vi "Adaptive ROI System.vi"() -> ()   [LabVIEW 2009]
uses:
  <vilib>/imath/engines/lvmath2/RunTimeEngine/ErrorHandling/NIMS_Finalize Error.vi
  <vilib>/imath/engines/lvmath2/RunTimeEngine/Parser/MC_Version.vi
  <vilib>/imath/engines/lvmath2/RunTimeEngine/NodeEndStatement/NIMS_NodeEndStatement_Output.vi
  <instcachedir>/0/NIMS_NodeEndStatement_Output_B70DDD75627E4997AAE11E9955EDAA25.lvgen/NIMS_NodeEndStatement_Output_B70DDD75627E4997AAE11E9955EDAA25_002.vi
  <instcachedir>/0/NIMS_NodeEndStatement_Output_B70DDD75627E4997AAE11E9955EDAA25.lvgen/NIMS_NodeEndStatement_Output_B70DDD75627E4997AAE11E9955EDAA25_001.vi
  <vilib>/imath/engines/lvmath/Functions/Error Handling/MergeErrorsWrapper.vi
  <vilib>/imath/engines/lvmath/Functions/Error Handling/error.ctl
  <vilib>/imath/engines/lvmath2/RunTimeEngine/BuiltInFunctions/abs/NIMS_abs(signed).vi
  <instcachedir>/0/NIMS_abs(signed)_C4FCB8E6058B49B797C7C8D53CA5F6EC.lvgen/NIMS_abs(signed)_C4FCB8E6058B49B797C7C8D53CA5F6EC_004.vi
  <instcachedir>/0/NIMS_NodeEndStatement_Output_B70DDD75627E4997AAE11E9955EDAA25.lvgen/NIMS_NodeEndStatement_Output_B70DDD75627E4997AAE11E9955EDAA25_006.vi
  <vilib>/imath/engines/lvmath/Functions/Error Handling/MC_Mask_Errors.vi
  <vilib>/imath/engines/lvmath2/RunTimeEngine/BuiltInFunctions/mean/NIMS_RRow=mean(RM,I32).vi
  <vilib>/imath/engines/lvmath2/RunTimeEngine/BuiltInFunctions/mean/NIMS_RS=mean(RV,I32).vi
  <vilib>/imathl/engines/lvmath/Functions/Error Handling/Create Error.vi
  <vilib>/imath/engines/lvmath2/RunTimeEngine/VariableToken/Read/NIMS_Get Elements - RV(_,_) - NoCheck - Check.vi
  <instcachedir>/0/NIMS_Get Elements - RV(_,_) - NoCheck - Check_2CF0E5988CCD4230910E4DE8A8D9652B.lvgen/NIMS_Get Elements - RV(_,_) - NoCheck - Check_2CF0E5988CCD4230910E4DE8A8D9652B_000.vi
  <vilib>/imath/engines/lvmath2/RunTimeEngine/RangeToken/NIMS_Range.vi
  <instcachedir>/0/NIMS_Range_6D647EC16A744C98B5DE1D649A2D648D.lvgen/NIMS_Range_6D647EC16A744C98B5DE1D649A2D648D_001.vi
  <vilib>/imath/engines/lvmath2/RunTimeEngine/VariableToken/Read/NIMS_Get Elements - RV(_) - Check(_).vi
  <instcachedir>/0/NIMS_Get Elements - RV(_) - Check(_)_82E0F2002B964B63A6FF4E3708911C3C.lvgen/NIMS_Get Elements - RV(_) - Check(_)_82E0F2002B964B63A6FF4E3708911C3C_000.vi
  <instcachedir>/0/NIMS_Range_6D647EC16A744C98B5DE1D649A2D648D.lvgen/NIMS_Range_6D647EC16A744C98B5DE1D649A2D648D_000.vi
  <vilib>/imath/engines/lvmath2/RunTimeEngine/BuiltInFunctions/max/1 input/NIMS_max(RV).vi
  <instcachedir>/0/NIMS_max(RV)_2C608606CE4049CAAC45B6670A7A9B83.lvgen/NIMS_max(RV)_2C608606CE4049CAAC45B6670A7A9B83_000.vi
  <vilib>/imath/engines/lvmath2/RunTimeEngine/BuiltInFunctions/is_nan/NIMS_is_nan.vi
  <instcachedir>/0/NIMS_is_nan_83F2CBA22B22468D9582265D5B29A05F.lvgen/NIMS_is_nan_83F2CBA22B22468D9582265D5B29A05F_000.vi
  <vilib>/imath/engines/lvmath2/RunTimeEngine/VariableToken/Read/NIMS_Get Elements - RV(_) - Check.vi
  <instcachedir>/0/NIMS_Get Elements - RV(_) - Check_60F12861D0564803969A5D0D0D1716CD.lvgen/NIMS_Get Elements - RV(_) - Check_60F12861D0564803969A5D0D0D1716CD_002.vi
  <vilib>/imath/engines/lvmath2/RunTimeEngine/ReplaceToken/NIMS_Replace - V(S)=S.vi
  <instcachedir>/0/NIMS_Replace - V(S)=S_670A9E0533664C1D848C8E58B3321B6A.lvgen/NIMS_Replace - V(S)=S_670A9E0533664C1D848C8E58B3321B6A_000.vi
  <vilib>/imath/engines/lvmath2/RunTimeEngine/ReplaceToken/NIMS_Replace - Size Check _(_)=S.vi
  <instcachedir>/0/NIMS_Replace - Size Check _(_)=S_8596181D73404097BAB9CBB006194BB0.lvgen/NIMS_Replace - Size Check _(_)=S_8596181D73404097BAB9CBB006194BB0_000.vi
  <vilib>/imath/engines/lvmath2/RunTimeEngine/ReplaceToken/NIMS_Replace - Check Linear.vi
  <instcachedir>/0/NIMS_Replace - Check Linear_9243CBB174894FF6977027453DA6955E.lvgen/NIMS_Replace - Check Linear_9243CBB174894FF6977027453DA6955E_001.vi
  <vilib>/imath/engines/lvmath2/RunTimeEngine/CommandStatement/MC_CommandStatement_break.vi
  <vilib>/imath/engines/lvmath2/RunTimeEngine/BuiltInFunctions/size/NIMS_[I32,I32]=size(GM).vi
  <instcachedir>/0/NIMS_[I32,I32]=size(GM)_B0A6EC1255BB4C8AB801FE6F734128D9.lvgen/NIMS_[I32,I32]=size(GM)_B0A6EC1255BB4C8AB801FE6F734128D9_000.vi
  <instcachedir>/0/NIMS_abs(signed)_C4FCB8E6058B49B797C7C8D53CA5F6EC.lvgen/NIMS_abs(signed)_C4FCB8E6058B49B797C7C8D53CA5F6EC_003.vi
  <vilib>/imath/engines/lvmath2/RunTimeEngine/VariableToken/NIMS_VariableToken_CondDefined.vi
  <instcachedir>/0/NIMS_VariableToken_CondDefined_5641E79000FB4D628475532441475385.lvgen/NIMS_VariableToken_CondDefined_5641E79000FB4D628475532441475385_000.vi
  <vilib>/imath/engines/lvmath2/RunTimeEngine/VariableToken/Read/NIMS_Get Elements - SorM(_,_) - Check(_) - Check(_).vi
  <instcachedir>/0/NIMS_Get Elements - SorM(_,_) - Check(_) - Check(_)_765307169EBF4B10AFB614967F0850B3.lvgen/NIMS_Get Elements - SorM(_,_) - Check(_) - Check(_)_765307169EBF4B10AFB614967F0850B3_000.vi
  <vilib>/imath/engines/lvmath/Functions/Error Handling/MC_Error Cluster From Error Code.vi
  <instcachedir>/0/NIMS_abs(signed)_C4FCB8E6058B49B797C7C8D53CA5F6EC.lvgen/NIMS_abs(signed)_C4FCB8E6058B49B797C7C8D53CA5F6EC_002.vi
  <vilib>/imath/engines/lvmath2/RunTimeEngine/BuiltInFunctions/fftshift/NIMS_fftshift(GM).vi
  <instcachedir>/0/NIMS_fftshift(GM)_854644D58B904BE68890FF38C728418A.lvgen/NIMS_fftshift(GM)_854644D58B904BE68890FF38C728418A_000.vi
  <vilib>/imath/engines/lvmath2/RunTimeEngine/BuiltInFunctions/fft2d/NIMS_fft2d.vi
  <instcachedir>/0/NIMS_fft2d_5F3590B2E5BC4AF3BD6395730A2DC379.lvgen/NIMS_fft2d_5F3590B2E5BC4AF3BD6395730A2DC379_000.vi
  <vilib>/imath/engines/lvmath2/RunTimeEngine/BuiltInFunctions/meshgrid2d/NIMS_meshgrid2d(V,V).vi
  <instcachedir>/0/NIMS_meshgrid2d(V,V)_E4FD91C5AC284970A2AC10945542E876.lvgen/NIMS_meshgrid2d(V,V)_E4FD91C5AC284970A2AC10945542E876_000.vi
  <vilib>/imath/engines/lvmath2/RunTimeEngine/BuiltInFunctions/cart_to_polar/NIMS_cart_to_polar(M3).vi
  <vilib>/imath/engines/lvmath2/RunTimeEngine/BuiltInFunctions/round/NIMS_round(DBL).vi
  <vilib>/imath/engines/lvmath2/RunTimeEngine/BuiltInFunctions/zeros/NIMS_V=zeros(I32,I32).vi
  <vilib>/imath/engines/lvmath2/RunTimeEngine/ReplaceToken/NIMS_Replace - Assignment Check _(_)=VorM.vi
  <instcachedir>/0/NIMS_Replace - Assignment Check _(_)=VorM_092AB1ED6AF9404A81BC0E556665BBDA.lvgen/NIMS_Replace - Assignment Check _(_)=VorM_092AB1ED6AF9404A81BC0E556665BBDA_001.vi
  <vilib>/imath/engines/lvmath2/RunTimeEngine/ReplaceToken/NIMS_Replace - Size Check _(_)=VorM.vi
  <instcachedir>/0/NIMS_Replace - Size Check _(_)=VorM_5D763D18DEEF46AFB676FCB035E69D92.lvgen/NIMS_Replace - Size Check _(_)=VorM_5D763D18DEEF46AFB676FCB035E69D92_001.vi
  <vilib>/imath/engines/lvmath2/RunTimeEngine/VariableToken/Read/NIMS_Get Elements - SorM(_) - Check.vi
  <instcachedir>/0/NIMS_Get Elements - SorM(_) - Check_7ED6A6929A794478AD00936E11BC64AA.lvgen/NIMS_Get Elements - SorM(_) - Check_7ED6A6929A794478AD00936E11BC64AA_000.vi
  <vilib>/imath/engines/lvmath2/RunTimeEngine/BuiltInFunctions/findnz/NIMS_[1o]_findnz(GM).vi
  <instcachedir>/0/NIMS_[1o]_findnz(GM)_DBE08F0D46E742F4956471D0BFAB2CB2.lvgen/NIMS_[1o]_findnz(GM)_DBE08F0D46E742F4956471D0BFAB2CB2_000.vi
  <instcachedir>/0/NIMS_Replace - Assignment Check _(_)=VorM_092AB1ED6AF9404A81BC0E556665BBDA.lvgen/NIMS_Replace - Assignment Check _(_)=VorM_092AB1ED6AF9404A81BC0E556665BBDA_000.vi
  <instcachedir>/0/NIMS_Replace - Size Check _(_)=VorM_5D763D18DEEF46AFB676FCB035E69D92.lvgen/NIMS_Replace - Size Check _(_)=VorM_5D763D18DEEF46AFB676FCB035E69D92_000.vi
  <instcachedir>/0/NIMS_Replace - Check Linear_9243CBB174894FF6977027453DA6955E.lvgen/NIMS_Replace - Check Linear_9243CBB174894FF6977027453DA6955E_000.vi
  <vilib>/imath/engines/lvmath2/RunTimeEngine/BuiltInFunctions/polyfit/NIMS_[2o]_polyfit.vi
  <vilib>/imath/engines/lvmath2/RunTimeSupport/NIMS_Complex To Real.vi
  <instcachedir>/0/NIMS_Complex To Real_7B9C6496820F433C8523AD0145A83A8A.lvgen/NIMS_Complex To Real_7B9C6496820F433C8523AD0145A83A8A_000.vi
  <vilib>/imath/engines/lvmath2/RunTimeEngine/VariableToken/NIMS_VariableToken_CondDefinedDefinedByReplace.vi
  <instcachedir>/0/NIMS_VariableToken_CondDefinedDefinedByReplace_D162CFFC24174562A9FEA619A91E1A56.lvgen/NIMS_VariableToken_CondDefinedDefinedByReplace_D162CFFC24174562A9FEA619A91E1A56_000.vi
  <instcachedir>/0/NIMS_abs(signed)_C4FCB8E6058B49B797C7C8D53CA5F6EC.lvgen/NIMS_abs(signed)_C4FCB8E6058B49B797C7C8D53CA5F6EC_001.vi
  <vilib>/imath/engines/lvmath2/RunTimeEngine/BuiltInFunctions/min/1 input/NIMS_min(RV).vi
  <instcachedir>/0/NIMS_min(RV)_AE994CF480B345CA9E0CB3DC5B6A3F66.lvgen/NIMS_min(RV)_AE994CF480B345CA9E0CB3DC5B6A3F66_000.vi
  <instcachedir>/0/NIMS_abs(signed)_C4FCB8E6058B49B797C7C8D53CA5F6EC.lvgen/NIMS_abs(signed)_C4FCB8E6058B49B797C7C8D53CA5F6EC_000.vi
  <vilib>/imath/engines/lvmath2/RunTimeEngine/BuiltInFunctions/rem/NIMS_rem_no checks.vi
  <instcachedir>/0/NIMS_rem_no checks_4CC9B305AB7E42EF90AFC4973FB32F8D.lvgen/NIMS_rem_no checks_4CC9B305AB7E42EF90AFC4973FB32F8D_000.vi
  <vilib>/imath/engines/lvmath2/RunTimeEngine/BuiltInFunctions/size/NIMS_I32Row=size(GM).vi
  <instcachedir>/0/NIMS_I32Row=size(GM)_10ACDCB9F1F84A7E9F42C91D87611FB5.lvgen/NIMS_I32Row=size(GM)_10ACDCB9F1F84A7E9F42C91D87611FB5_000.vi
  <instcachedir>/0/NIMS_NodeEndStatement_Output_B70DDD75627E4997AAE11E9955EDAA25.lvgen/NIMS_NodeEndStatement_Output_B70DDD75627E4997AAE11E9955EDAA25_005.vi
  <instcachedir>/0/NIMS_Get Elements - RV(_) - Check_60F12861D0564803969A5D0D0D1716CD.lvgen/NIMS_Get Elements - RV(_) - Check_60F12861D0564803969A5D0D0D1716CD_001.vi
  <vilib>/imath/engines/lvmath2/RunTimeEngine/BuiltInFunctions/conv2d/NIMS_conv2d(GM,GM,Str).vi
  <instcachedir>/0/NIMS_conv2d(GM,GM,Str)_C7D81E1B98E043D08C3460674E88E962.lvgen/NIMS_conv2d(GM,GM,Str)_C7D81E1B98E043D08C3460674E88E962_001.vi
  <vilib>/imath/engines/lvmath2/RunTimeEngine/ArithmeticOperatorToken/NIMS_ArithmeticOperator_plus.vi
  <instcachedir>/0/NIMS_ArithmeticOperator_plus_C2557ADBC1AF4CC89A8D103312A7892D.lvgen/NIMS_ArithmeticOperator_plus_C2557ADBC1AF4CC89A8D103312A7892D_002.vi
  <vilib>/imath/engines/lvmath2/RunTimeEngine/BuiltInFunctions/sum/NIMS_sum(GM,Sca).vi
  <instcachedir>/0/NIMS_sum(GM,Sca)_1EB0DF48B4224309BC0660E7CC5423AB.lvgen/NIMS_sum(GM,Sca)_1EB0DF48B4224309BC0660E7CC5423AB_000.vi
  <vilib>/imath/engines/lvmath2/RunTimeEngine/VariableToken/Read/NIMS_Get Elements - SorM(_,_) - Check - Check.vi
  <instcachedir>/0/NIMS_Get Elements - SorM(_,_) - Check - Check_48F983ECF9704C8392806B5FDD2F5E51.lvgen/NIMS_Get Elements - SorM(_,_) - Check - Check_48F983ECF9704C8392806B5FDD2F5E51_001.vi
  <vilib>/imath/engines/lvmath2/RunTimeEngine/BuiltInFunctions/sum/NIMS_sum(GV).vi
  <instcachedir>/0/NIMS_sum(GV)_6582ACC3CFD94C22B1CA3BD4A8C5E9ED.lvgen/NIMS_sum(GV)_6582ACC3CFD94C22B1CA3BD4A8C5E9ED_000.vi
  <instcachedir>/0/NIMS_Get Elements - RV(_) - Check_60F12861D0564803969A5D0D0D1716CD.lvgen/NIMS_Get Elements - RV(_) - Check_60F12861D0564803969A5D0D0D1716CD_000.vi
  <vilib>/imath/engines/lvmath2/RunTimeEngine/VariableToken/Read/NIMS_Get Elements - CV(_) - Check.vi
  <instcachedir>/0/NIMS_Get Elements - CV(_) - Check_BEC96A94B22A447C8D443292564CBCD4.lvgen/NIMS_Get Elements - CV(_) - Check_BEC96A94B22A447C8D443292564CBCD4_000.vi
  <vilib>/imath/engines/lvmath2/RunTimeEngine/ReplaceToken/NIMS_Replace - M(#,S)=S.vi
  <instcachedir>/0/NIMS_Replace - M(#,S)=S_1219E6139A4243FF9F5238A5EFF7E472.lvgen/NIMS_Replace - M(#,S)=S_1219E6139A4243FF9F5238A5EFF7E472_001.vi
  <vilib>/imath/engines/lvmath2/RunTimeEngine/ReplaceToken/NIMS_Replace - Size Check M(#,_)=S.vi
  <instcachedir>/0/NIMS_Replace - Size Check M(#,_)=S_E9F0A723BCFB4C07851EF854435358BF.lvgen/NIMS_Replace - Size Check M(#,_)=S_E9F0A723BCFB4C07851EF854435358BF_001.vi
  <vilib>/imath/engines/lvmath2/RunTimeEngine/ReplaceToken/NIMS_Replace - Check(_) Column.vi
  <instcachedir>/0/NIMS_Replace - Check(_) Column_2F70AC15C33C40AE8160DC5A87C7C261.lvgen/NIMS_Replace - Check(_) Column_2F70AC15C33C40AE8160DC5A87C7C261_003.vi
  <vilib>/imath/engines/lvmath2/RunTimeEngine/Managers/WorkSpace/UID Generator.vi
  <instcachedir>/0/NIMS_NodeEndStatement_Output_B70DDD75627E4997AAE11E9955EDAA25.lvgen/NIMS_NodeEndStatement_Output_B70DDD75627E4997AAE11E9955EDAA25_007.vi
  <vilib>/imath/engines/lvmath2/RunTimeEngine/Managers/SymbolTable/Clear UID.vi
  <vilib>/imath/engines/lvmath2/RunTimeEngine/LocalVariableDefStatement/MC_LocalVariableDefStatement_Display.vi
  <vilib>/imath/engines/lvmath2/RunTimeEngine/RunTimeType/NIMS_RunTimeType_From StrictType (excl LVString).vi
  <instcachedir>/0/NIMS_ArithmeticOperator_plus_C2557ADBC1AF4CC89A8D103312A7892D.lvgen/NIMS_ArithmeticOperator_plus_C2557ADBC1AF4CC89A8D103312A7892D_001.vi
  <vilib>/imath/engines/lvmath2/RunTimeEngine/VariableToken/Read/NIMS_Get Elements - SorM(#,_) - Check(_).vi
  <instcachedir>/0/NIMS_Get Elements - SorM(#,_) - Check(_)_3C902678D53E40FDBC79E118A936F6E4.lvgen/NIMS_Get Elements - SorM(#,_) - Check(_)_3C902678D53E40FDBC79E118A936F6E4_000.vi
  <vilib>/vision/NI_Vision_Development_Module.lvlib
  <vilib>/imath/engines/lvmath2/RunTimeEngine/Managers/SymbolTable/NIMS_WorkSpace.lvlib
panel:
  in  "AVI file to play":path
  out "focus":dbl[](array[numeric])
  out "edge":dbl[](array[numeric])
  out "motion":dbl[](array[numeric])
  out "Frame #":dbl
  out "Edge Detectives 2":dbl[](array[numeric])
  out "Image 4":T1(plugin-control)
  in  "Threshold 2":dbl=125.0
  out "Image 2":T1(plugin-control)
  in  "% thru movie":dbl(slide) scale=0.0..95.0
  out "Frame Width":dbl
  out "Frame height":dbl
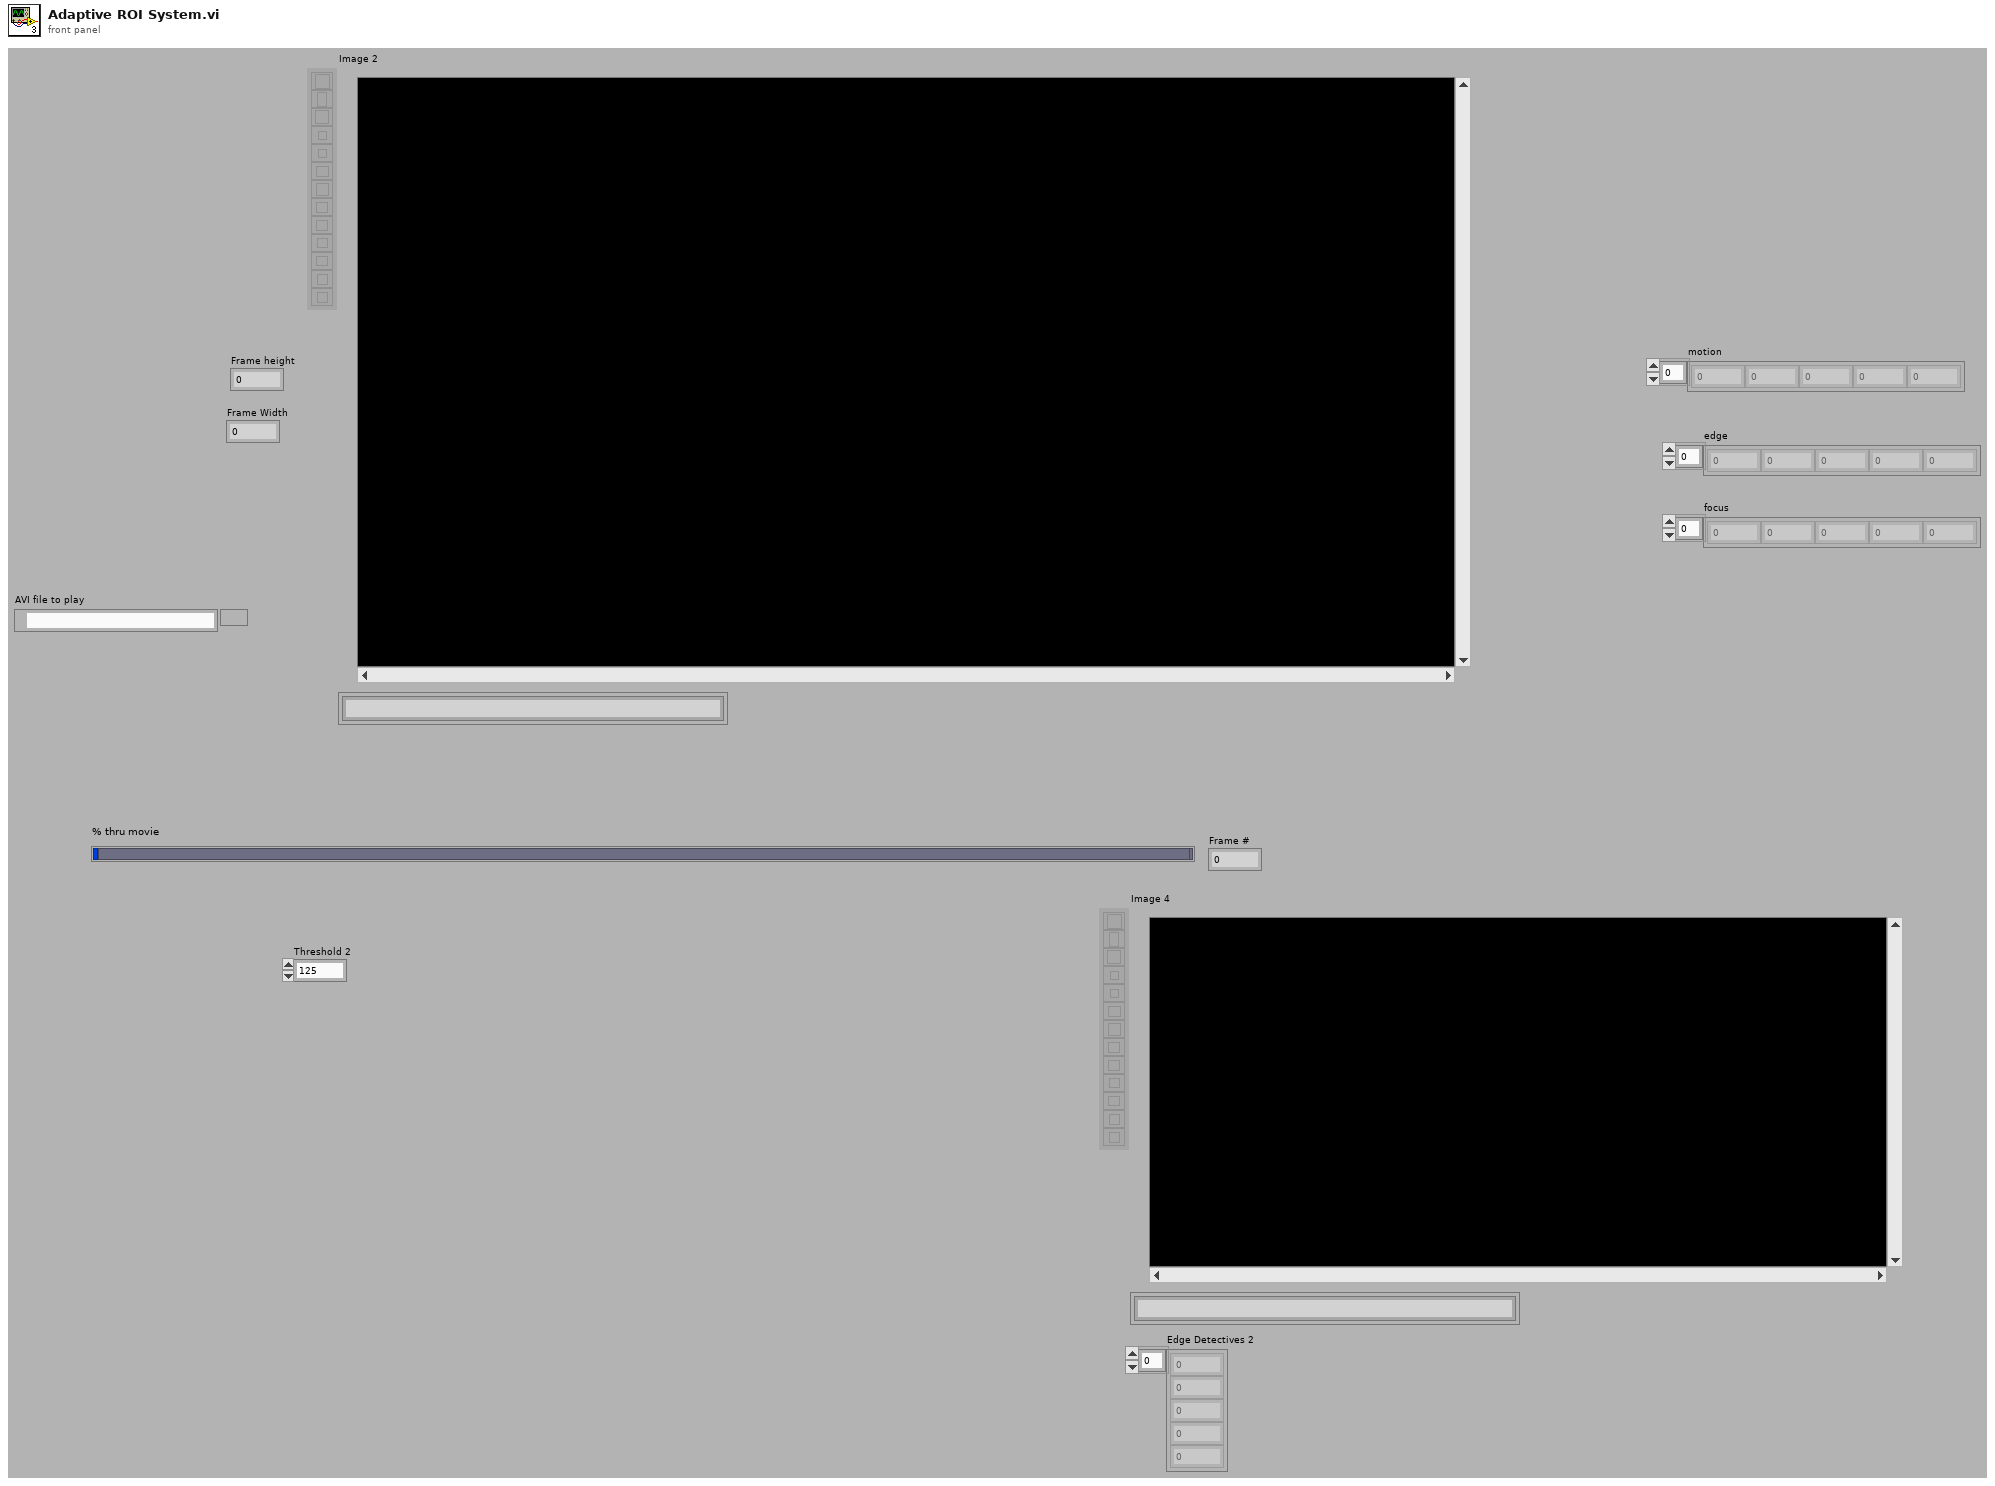
[diagram p1: front panel]
types:
  T1 = typedef "IMAQ Image.ctl" = refnum<image>
  T2 = typedef "AviRefnum.ctl" = refnum<k1>
  T3 = typedef "Image Type" = u32
  T4 = cluster{"width":u32, "height":u32, "framesPerSecond":u32, "compressionFilter":string, "hasData":bool}
  T5 = typedef "error.ctl" = enum16{"No Error", "Problem", "Unused002", "Incorrect number of parameters", "Function not defined for non-numeric types", "Unused005", "Function only defined for character arrays", "Function not defined for boolean, character, or single precision", "Function not defined for complex types", "Not a valid operation", "Inputs must be scalar", "Input matrices are not the same size", "Unused012", "Input matrices must be nonnegative integers of the same type", "Arguments must be non-negative integers less than bitmax", "Number to complement must be less than 2^N", "Bit to get is outside range", "Bit to set is outside range", "Input must be real type ", "At least one parameter must be scalar", "Unused020", "Function not defined for\nhigher dimensional matrices.", "Invalid attributes", "Wrong Type of Input Arguments", "Wrong Argument Option", "Unused025", "Indices must be real positive integers", "Unused027", "Number of elements must be the same for indices and values", "Unused029", "Cannot resize a 2D matrix with a linear index", "Unknown variable or symbol", "Indices out of range", "Empty matrix deletion can not be used with two indices", "Number of rows and columns must be the same for indices and values.", "Complex cannot be converted to Boolean", "Char cannot be converted to Boolean", "int64 cannot be converted to Boolean", "uint64 cannot be converted to Boolean", "Unused039", "Unused040", "All rows must have the same number of columns", "Incompatible types", "Invalid matrix dimensions", "Dimension must be 1 or 2", "Base must be an integer between 2 and 36", "Invalid input", "Square matrix required", "Function 'timerstart' must be called before 'timerstop'", "Arguments must be positive real", "Step must not be zero", "Wrong number of input arguments", "Wrong number of output arguments", "Unused053", "Input scalar must be >= 0", "Input scalar must be positive", "Input scalar must not be 0", "Input scalar must be in range [0,1]", "Unused058", "Input must be a vector", "Unused060", "Empty vector error", "All elements must be in domain [-1,1]", "All real elements of input vector must be >= 0", "All elements of input vector must be positive", "Values of input vectors are not compatible", "Unused066", "Input vector must be an increasing vector", "Unused068", "Unused069", "Lenths of two input vectors are not compatible", "Unused071", "Empty matrix error", "Unused073", "Unused074", "Unused075", "Unused076", "Unused077", "Size of input matrix is incompatible with input size", "Invalid format specifier", "Unused080", "Unused081", "Unused082", "Unused083", "Unused084", "Unused085", "RunTime: MathScript could not be compiled", "Unknown function", "Only scalars and strings supported", "Unused089", "Unused090", "Range is too large", "End used without variable", "Function not available (RTE)", "Custom user error", "Arguments must be integers less than bitmax", "Shared library not found", "Header file not found", "Shared library already loaded", "Shared library not loaded", "Shared library function not found", "Shared library string return problem", "Problem calling shared library function", "Problem loading shared library from OS", "Problem parsing shared library header file", "Shared library incompatible types", "Shared library unsupported return type", "Shared library function not exported", "Shared library unsupported input type", "Problem unloading shared library from OS", "Function only available from UI", "Invalid function specified in argument", "An internal error has occurred", "Invalid object", "Invalid property", "Read-only property", "A break command has occurred", "A continue command has occurred", "A return command has occurred", "ode: times parameter invalid", "Unused120", "Function not found in file", "Reserved keyword cannot be defined as variable", "Reserved keyword cannot be defined as a function or script", "Arguments must be string literals", "Function not supported on this platform", "All columns must have the same number of rows", "Function ignored in RTE warning", "Cannot use : as a parameter that is not a variable", "Output can't be coerced to requested type", "Function not supported on current target", "Variable dependent on an unwired function input", "Unused132", "Unused133", "Unused134", "Unused135", "Unused136", "Unused137", "Unused138", "Unused139", "Unused140", "Unused141", "Unused142", "Unused143", "Unused144", "Unused145", "Unused146", "MathScript parser DLL missing", "MathScript requires LabVIEW Full", "MathScript license is invalid or missing"}
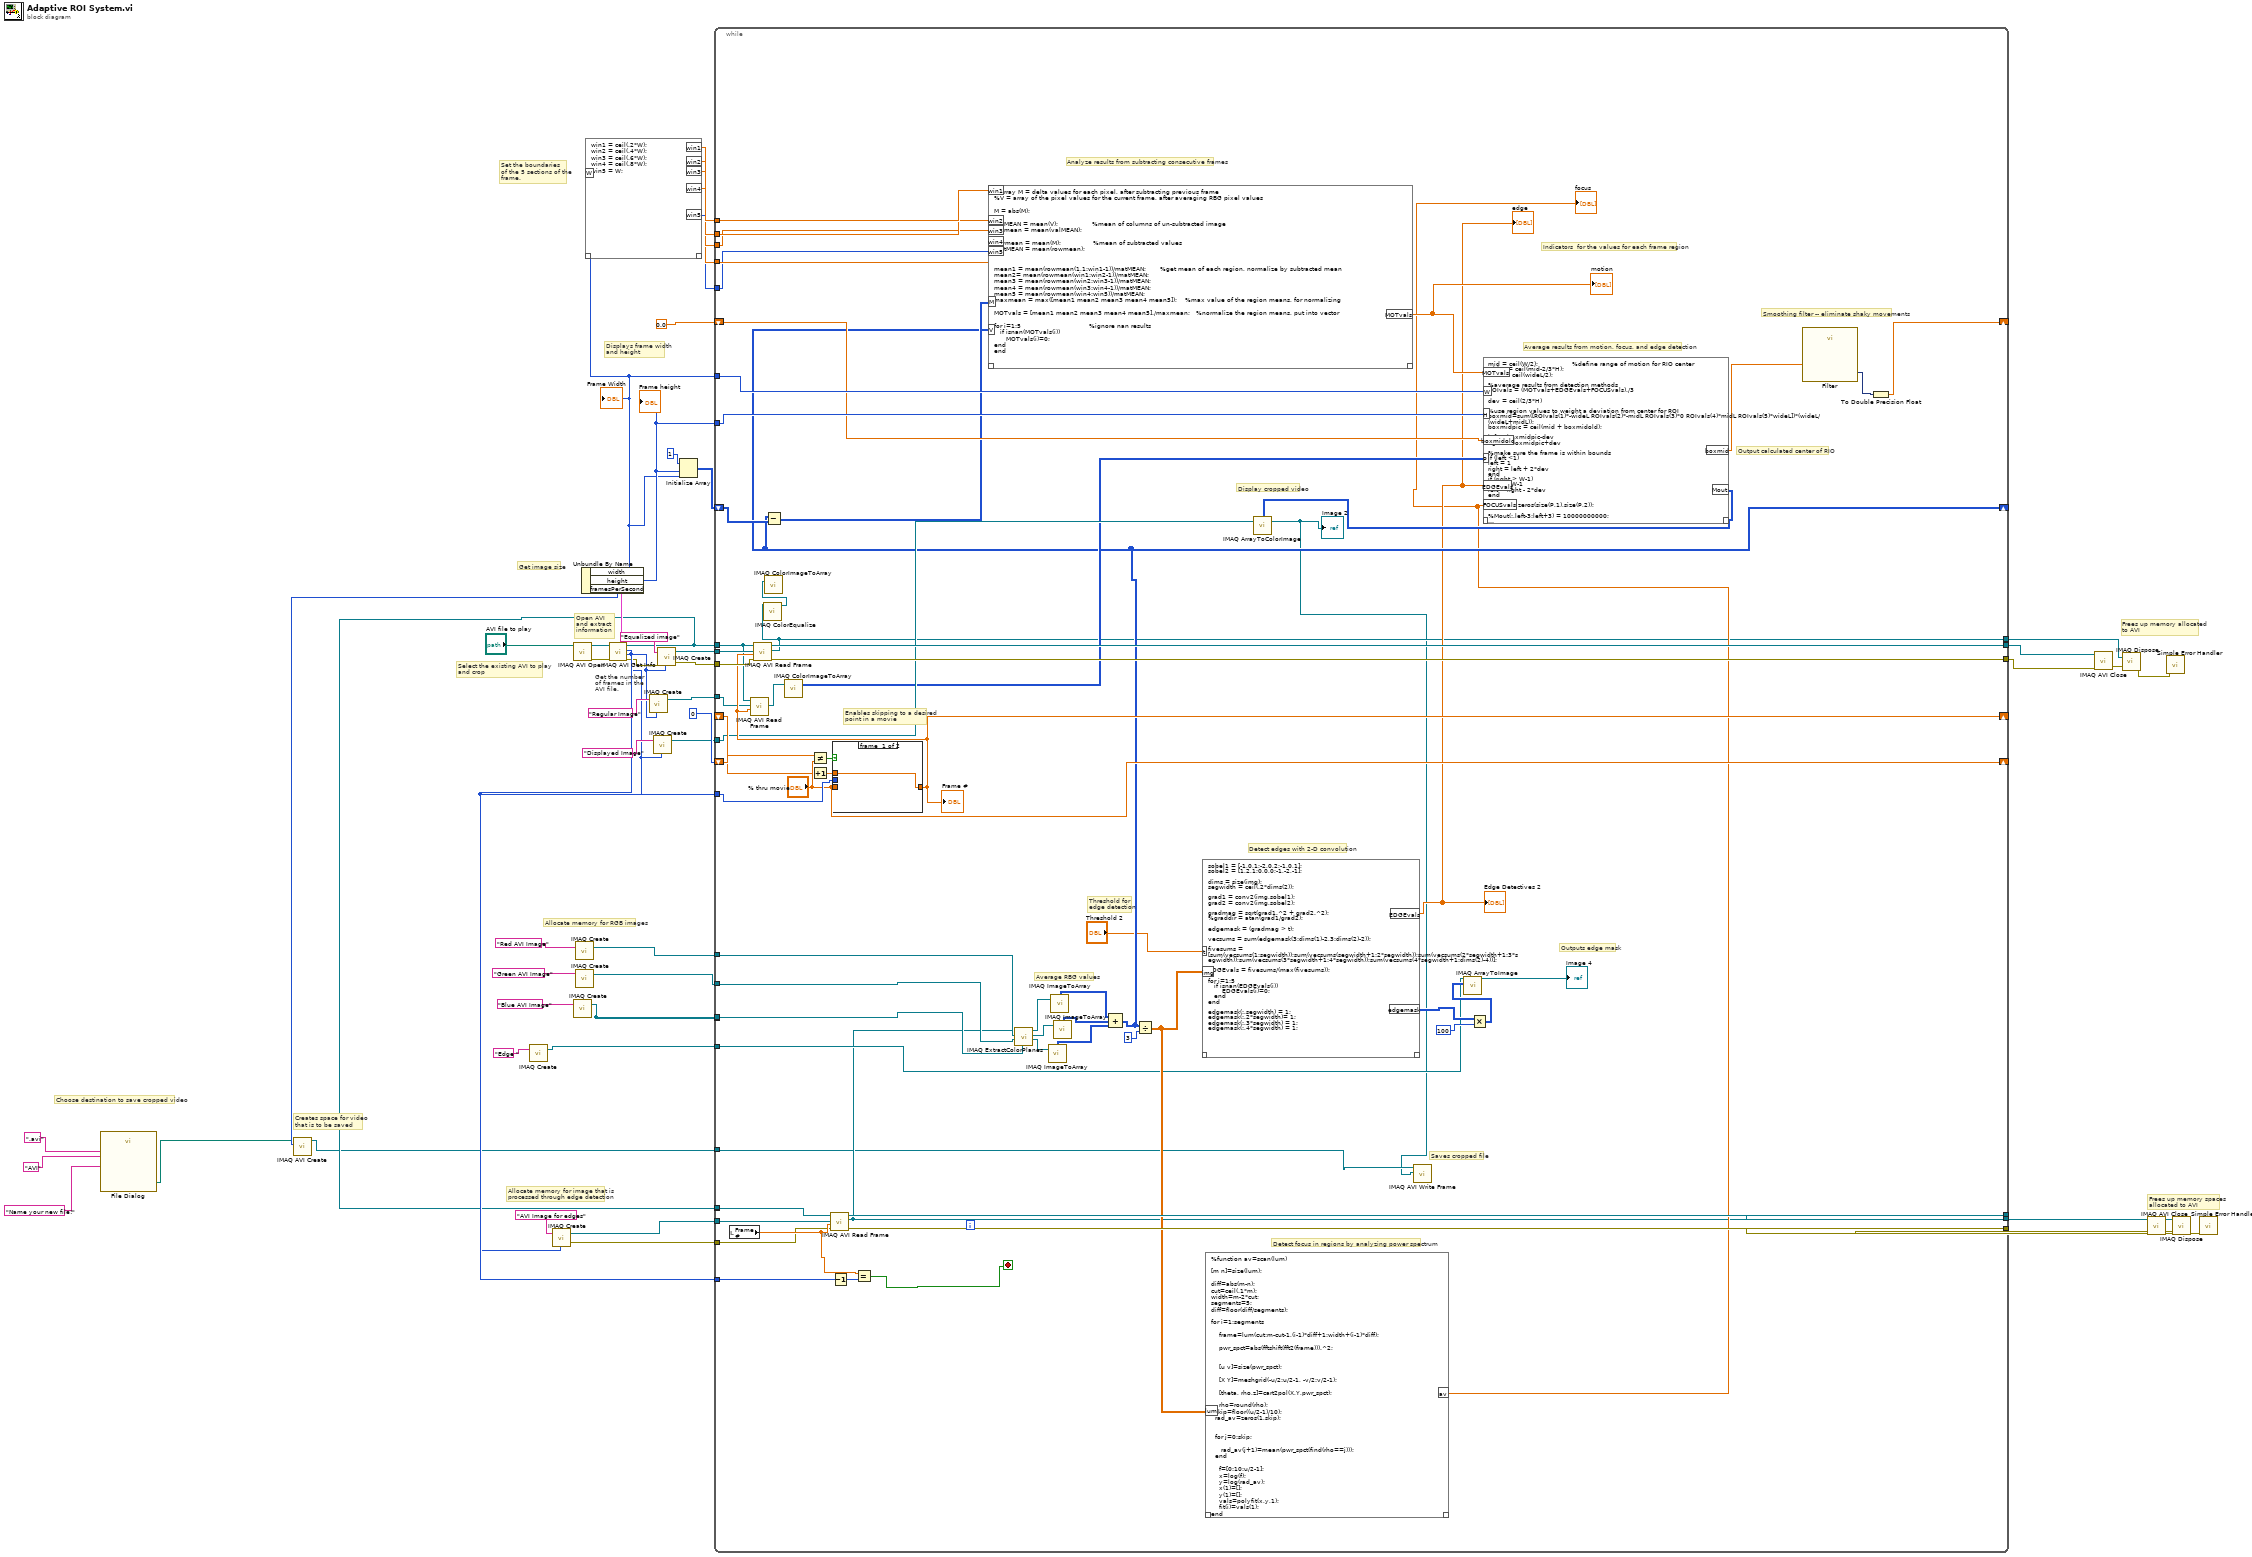
[diagram p0: block diagram]
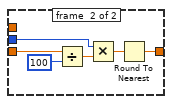
[diagram p2: hidden frame]
diagram:
  # "Creates space for video\nthat is to be saved"
  # "Displays frame width\nand height"
  # "Frees up memory allocated\nto AVI"
  # "Frees up memory spaces\nallocated to AVI"
  # "Open AVI and extract information"
  # "Allocate memory for image that is \nprocessed through edge detection"
  # "Get image size"
  # "Set the boundaries\nof the 5 sections of the\nframe."
  # "Select the existing AVI to play\nand crop"
  # "Allocate memory for RGB images"
  # "Choose destination to save cropped video"
  # "Get the number\nof frames in the\nAVI file."
  n1 = call "File Dialog"("prompt"="Name your new file!", "pattern (all files)"=".avi", "pattern label"="AVI") -> ("selected path"=w2:path)  [unwired: 9 in, 3 out]
  n2 = call "IMAQ Create"("Image Name"="Edge ") -> ("New Image"=w21:T1)  [unwired: 4 in, 1 out]
  n3 = call "IMAQ AVI Open"("AVI Path"="AVI file to play") -> ("error out"=w50:errorcluster, "Avi Refnum"=w49:T2)  [unwired: 1 in, 8 out]
  n4 = call "IMAQ Create"("Image Name"="Blue AVI Image") -> ("New Image"=w22:T1)  [unwired: 4 in, 1 out]
  n5 = call "IMAQ Create"("Image Name"="Red AVI Image") -> ("New Image"=w24:T1)  [unwired: 4 in, 1 out]
  n6 = call "IMAQ Create"("Image Name"="Green AVI Image") -> ("New Image"=w23:T1)  [unwired: 4 in, 1 out]
  n7 = call "IMAQ AVI Get Info"("error in (no error)"=w50, "Avi Refnum"=w49) -> ("error out"=w4:errorcluster, "Image Type"=w3:T3, "Number of Frames"=w20:u32, "Avi Refnum (duplicate)"=w18:T2, "Frame Data"=w51:T4)  [unwired: 5 out]
  n8 = call "IMAQ Create"("Image Name"="AVI Image for edges", "Image Type"=w3) -> ("New Image"=w19:T1, "error out"=w16:errorcluster)  [unwired: 2 in, 1 out]
  n9 = Unbundle By Name(w51) -> ("width"=w30:u32, "height"=w36:u32, "framesPerSecond"=w5:u32)
  "Frame height" <- w36
  "Frame Width" <- w30
  n10 = call "IMAQ AVI Create"("Frames Per Second"=w5, "AVI Path"=w2) -> ("Avi Refnum"=w11:T2)  [unwired: 8 in, 1 out]
  n11 = mathscript code="win1 = ceil(.2*W);\nwin2 = ceil(.4*W);\nwin3 = ceil(.6*W);\nwin4 = ceil(.8*W);\nwin5 = W;"("W"=w30) -> ("win1"=w35:dbl, "win2"=w34:dbl, "win3"=w33:dbl, "win4"=w32:dbl, "win5"=w31:u32)  [unwired: 1 in, 1 out]
  n12 = call "IMAQ Create"("Image Name"="Regular Image", "Image Type"=w3) -> ("New Image"=w39:T1)  [unwired: 3 in, 1 out]
  n13 = call "IMAQ Create"("Image Name"="Displayed Image", "Image Type"=w3) -> ("New Image"=w37:T1)  [unwired: 3 in, 1 out]
  n14 = call "IMAQ Create"("Image Name"="Equalized image", "Image Type"=w3, "error in (no error)"=w4) -> ("New Image"=w46:T1, "error out"=w15:errorcluster)  [unwired: 1 in, 1 out]
  n15 = Initialize Array(1, w36, w30) -> (w42:i32[][])
  n16 = while {
    tunnel: w46 -> [w117]
    tunnel: [w118] -> w47
    tunnel: [w116] -> w48
    tunnel: w18 -> [w106]
    tunnel: [w61] -> w44
    tunnel: w15 -> [w115]
    shift-right: [w68] -> _
    shift-left: w42 -> [w108]
    tunnel: w20 -> [w112]
    shift-right: ["% thru movie"] -> _
    shift-left: 0 -> [w114]
    shift-right: [w107] -> _
    shift-left: _ -> [w110]
    tunnel: w39 -> [w60]
    tunnel: w37 -> [w105]
    tunnel: w30 -> [w74]
    tunnel: w36 -> [w73]
    tunnel: w35 -> [w104]
    tunnel: w34 -> [w103]
    tunnel: w33 -> [w102]
    tunnel: w32 -> [w101]
    tunnel: w31 -> [w100]
    shift-right: [w98] -> _
    shift-left: 0.0 -> [w72]
    tunnel: w24 -> [w87]
    tunnel: w23 -> [w86]
    tunnel: w22 -> [_]
    tunnel: w22 -> [w85]
    tunnel: w21 -> [w58]
    tunnel: w20 -> [w83]
    tunnel: w19 -> [w80]
    tunnel: [w79] -> _
    tunnel: w18 -> [w79]
    tunnel: w16 -> [w78]
    tunnel: w11 -> [w55]
    tunnel: [w77] -> w10
    tunnel: [w57] -> w8
    tunnel: [w76] -> w9
    stop <- w81 stop-if-true
    # "Threshold for \nedge detection"
    # "Enables skipping to a desired\npoint in a movie"
    # "Saves cropped file"
    # "Outputs edge mask"
    # "Detect focus in regions by analyzing power spectrum"
    # "Average RBG values"
    # "Detect edges with 2-D convolution"
    # "Display cropped video"
    # "Output calculated center of RIO"
    # "Average results from motion, focus, and edge detection"
    # "Smoothing filter -- eliminate shaky movements"
    # "Indicators  for the values for each frame region"
    # "Analyze results from subtracting consecutive frames"
    n17 = local read "Frame #"() -> (w82:dbl)
    n18 = Not Equal?(x=w114, y="% thru movie") -> (x != y?=w113:bool)
    n19 = Increment(x=w110) -> (x+1=w109:dbl)
    n20 = call "IMAQ AVI Read Frame"("error in (no error)"=w78, "Frame Number"=w82, "Image"=w80, "Avi Refnum"=w79) -> ("error out"=w77:errorcluster, "Image Out"=w57:T1, "Avi Refnum (duplicate)"=w76:T2)  [unwired: 1 in, 4 out]
    n21 = Decrement(x=w83) -> (x-1=w84:u32)
    n22 = case shown="True" w113 {
      tunnel: "% thru movie" -> [_ w1788]
      tunnel: w112 -> [_ w1791]
      tunnel: [w1785 w1789] -> w107
      tunnel: w109 -> [w1785 _]
      frame #0 {
      }
      frame #1 {
        n23 = Divide(x=w1788, y=100) -> (x/y=w1786:dbl)
        n24 = Multiply(x=w1791, y=w1786) -> (x*y=w1790:dbl)
        n25 = Round To Nearest(number=w1790) -> (nearest integer value=w1789:dbl)
      }
    }
    "Frame #" <- w107
    n26 = call "IMAQ AVI Read Frame"("Frame Number"=w107, "Image"=w60, "Avi Refnum"=w106) -> ("Image Out"=w56:T1)  [unwired: 2 in, 6 out]
    n27 = call "IMAQ AVI Read Frame"("error in (no error)"=w115, "Frame Number"=w107, "Image"=w117, "Avi Refnum"=w106) -> ("error out"=w116:errorcluster, "Image Out"=w61:T1, "Avi Refnum (duplicate)"=w118:T2)  [unwired: 1 in, 4 out]
    n28 = call "IMAQ ColorEqualize"("Image Src"=w61) -> ("Image Dst Out"=w75:T1)  [unwired: 4 in, 1 out]
    n29 = call "IMAQ ColorImageToArray"("Image"=w75) -> ()  [unwired: 3 in, 3 out]
    n30 = call "IMAQ ColorImageToArray"("Image"=w56) -> ("Image Pixels (U32)"=w70:u32[][])  [unwired: 3 in, 2 out]
    n31 = Equal?(x=w82, y=w84) -> (x = y?=w81:bool)
    n32 = call "IMAQ ExtractColorPlanes"("Blue or Luma or Val or Inten Plane"=w85, "Green or Sat Plane"=w86, "Red or Hue Plane"=w87, "Image Src"=w57) -> ("Blue or Luma or Val or Inten Plane out"=w95:T1, "Green or Sat Plane out"=w96:T1, "Red or Hue Plane out"=w97:T1)  [unwired: 4 in, 1 out]
    n33 = call "IMAQ ImageToArray"("Image"=w95) -> ("Image Pixels (U8)"=w92:u8[][])  [unwired: 3 in, 4 out]
    n34 = call "IMAQ ImageToArray"("Image"=w97) -> ("Image Pixels (U8)"=w94:u8[][])  [unwired: 3 in, 4 out]
    n35 = call "IMAQ ImageToArray"("Image"=w96) -> ("Image Pixels (U8)"=w93:u8[][])  [unwired: 3 in, 4 out]
    n36 = Compound Arithmetic op=ADD(w94, w93, w92) -> (w68:u8[][])
    n37 = Subtract(x=w68, y=w108) -> (x-y=w69:i32[][])
    n38 = mathscript code="%array M = delta values for each pixel, after subtracting previous frame\n%V = array of the pixel values for the current frame, after averaging RBG pixel values\n\nM = abs(M);\n\nvalMEAN = mean(V);                 %mean of columns of un-subtracted image\nvalmean = mean(valMEAN);\n         \nrowmean = mean(M);                %mean of subtracted values\nmatMEAN = mean(rowmean);\n\n\nmean1 = mean(rowmean(1,1:win1-1))/matMEAN;       %get mean of each region, normalize by subtracted mean\nmean2= mean(rowmean(win1:win2-1))/matMEAN;\nmean3 = mean(rowmean(win2:win3-1))/matMEAN;\nmean4 = mean(rowmean(win3:win4-1))/matMEAN;\nmean5 = mean(rowmean(win4:win5))/matMEAN;\nmaxmean = max([mean1 mean2 mean3 mean4 mean5]);    %max value of the region means, for normalizing\n\nMOTvals = [mean1 mean2 mean3 mean4 mean5]./maxmean;   %normalize the region means, put into vector\n\nfor i=1:5                                  %ignore nan results\n   if isnan(MOTvals(i))\n      MOTvals(i)=0;\nend\nend"("M"=w69, "V"=w68, "win1"=w104, "win2"=w103, "win3"=w102, "win4"=w101, "win5"=w100) -> ("MOTvals"=w65:dbl[])  [unwired: 1 in, 1 out]
    "motion" <- w65
    n39 = Divide(x=w68, y=3) -> (x/y=w66:dbl[][])
    n40 = mathscript code="sobel1 = [-1,0,1;-2,0,2;-1,0,1];\nsobel2 = [1,2,1;0,0,0;-1,-2,-1];\n\ndims = size(img);\nsegwidth = ceil(.2*dims(2));\n\ngrad1 = conv2(img,sobel1);\ngrad2 = conv2(img,sobel2);\n\ngradmag = sqrt(grad1.^2 + grad2.^2);\n%graddir = atan(grad1/grad2);\n\nedgemask = (gradmag > t);\n\nvecsums = sum(edgemask(3:dims(1)-2,3:dims(2)-2));\n\nfivesums = [sum(vecsums(1:segwidth));sum(vecsums(segwidth+1:2*segwidth));sum(vecsums(2*segwidth+1:3*segwidth));sum(vecsums(3*segwidth+1:4*segwidth));sum(vecsums(4*segwidth+1:dims(2)-4))];\n\nEDGEvals = fivesums/(max(fivesums));\n\nfor i=1:5\n   if isnan(EDGEvals(i))\n       EDGEvals(i)=0;\n   end\nend\n\nedgemask(:,segwidth) = 1;\nedgemask(:,2*segwidth)= 1;\nedgemask(:,3*segwidth) = 1;\nedgemask(:,4*segwidth) = 1;"("img"=w66, "t"="Threshold 2") -> ("edgemask"=w88:i32[][], "EDGEvals"=w64:dbl[])  [unwired: 1 in, 1 out]
    "Edge Detectives 2" <- w64
    "edge" <- w64
    n41 = mathscript code="%function av=scan(lum)\n\n[m n]=size(lum);\n\ndiff=abs(m-n);\ncut=ceil(.1*m);\nwidth=m-2*cut;\nsegments=5;\ndiff=floor(diff/segments);\n\nfor i=1:segments\n  \n    frame=lum(cut:m-cut-1,(i-1)*diff+1:width+(i-1)*diff);\n\n    pwr_spct=abs(fftshift(fft2(frame))).^2;\n\n    \n    [u v]=size(pwr_spct);\n\n    [X Y]=meshgrid(-u/2:u/2-1, -v/2:v/2-1);\n\n    [theta, rho,z]=cart2pol(X,Y,pwr_spct);\n\n    rho=round(rho);\n  skip=floor((u/2-1)/10);\n  rad_av=zeros(1,skip);\n  \n\n  for j=0:skip;\n      \n     rad_av(j+1)=mean(pwr_spct(find(rho==j)));\n  end\n   \n    f=[0:10:u/2-1];\n    x=log(f);\n    y=log(rad_av);\n    x(1)=[];\n    y(1)=[];\n    vals=polyfit(x,y,1);\n    fit(i)=vals(1);\nend\n\n\nraw=fit;\n\nfor i=1:segments\n    fit(i)=abs(abs(fit(i))-2);\nend \n\n\nfor i=1:segments\n    fit(i)=fit(i)-min(fit);\nend\n\nfit=fit./max(fit);\n\nfit=abs(fit-1);\n%fit=fit./max(fit);\n\n%fit=abs(fit-1);\n%fit=fit./max(fit);\n\nr=rem(segments,5);\n\nl=(segments-r)/5;\n\nfor i=1:segments\n    if isnan(fit(i))\n        fit(i)=0;\n    end\nend\n\nfor i=1:5;\n   av(i)=mean(fit((i-1)*l+1:i*l));\nend"("lum"=w66) -> ("av"=w63:dbl[])  [unwired: 1 in, 1 out]
    "focus" <- w63
    n42 = Multiply(x=w88, y=100) -> (x*y=w89:i32[][])
    n43 = call "IMAQ ArrayToImage"("Image Pixels (U8)"=w89, "Image"=w58) -> ("Image Out"=→"Image 4":T1)  [unwired: 8 in, 1 out]
    n44 = mathscript code="mid = ceil(W/2);                 %define range of motion for RIO center\nwideL = ceil(mid-2/3*H);\nmidL = ceil(wideL/2);\n\n%average results from detection methods\nROIvals = (MOTvals+EDGEvals+FOCUSvals)./3\n\ndev = ceil(2/3*H)\n\n%use region values to weight a deviation from center for ROI\nboxmid=sum([ROIvals(1)*-wideL ROIvals(2)*-midL ROIvals(3)*0 ROIvals(4)*midL ROIvals(5)*wideL])*(wideL/(wideL+midL)); \nboxmidpic = ceil(mid + boxmidold);\n\nleft = boxmidpic-dev\nright = boxmidpic+dev\n\n%make sure the frame is within bounds\nif (left <1)\nleft = 1\nright = left + 2*dev\nend\nif (right > W-1)\nright = W-1\nleft = right - 2*dev\nend\n\n%Mout = zeros(size(P,1),size(P,2));\n\n%Mout(:,left-3:left+3) = 10000000000;\n\n%Mout(:,right-3:right+3) = 10000000000;\n\n%P is un-processed image array\nMout = P(:,left:right);  %output cropped image"("W"=w74, "H"=w73, "MOTvals"=w65, "boxmidold"=w72, "P"=w70, "EDGEvals"=w64, "FOCUSvals"=w63) -> ("boxmid"=w71:dbl, "Mout"=w67:u32[][])  [unwired: 1 in, 1 out]
    n45 = call "IMAQ ArrayToColorImage"("Image Pixels (U32)"=w67, "Image"=w105) -> ("Image Out"=w54:T1)  [unwired: 3 in, 1 out]
    "Image 2" <- w54
    n46 = call "IMAQ AVI Write Frame"("Image"=w54, "Avi Refnum"=w55) -> ()  [unwired: 8 in, 2 out]
    n47 = call "Filter"("Signal"=w71) -> ("Filtered Signal"=w99:dynamicdata)  [unwired: 9 in, 1 out]
    n48 = To Double Precision Float(number=w99) -> (double precision float=w98:dbl)
  }
  n49 = call "IMAQ AVI Close"("error in (no error)"=w48, "Avi Refnum"=w47) -> ("error out"=w45:errorcluster)  [unwired: 9 out]
  n50 = call "IMAQ Dispose"("Image"=w44, "error in (no error)"=w45) -> ("error out"=w52:errorcluster)  [unwired: 1 in, 3 out]
  n51 = call "IMAQ AVI Close"("error in (no error)"=w10, "Avi Refnum"=w9) -> ("error out"=w7:errorcluster)  [unwired: 9 out]
  n52 = call <vilib>:"Simple Error Handler.vi"("error in (no error)"=w52) -> ()  [unwired: 1 in, 8 out]
  n53 = call "IMAQ Dispose"("Image"=w8, "error in (no error)"=w7) -> ("error out"=w6:errorcluster)  [unwired: 1 in, 3 out]
  n54 = call <vilib>:"Simple Error Handler.vi"("error in (no error)"=w6) -> ()  [unwired: 1 in, 8 out]
